vi "SetDG with FileParamters.vi"(8 "error in (no error)":errorcluster, 10 "State":T1, 11 "BME_DG_Base in":refnum<class "BME_DG_Base.lvclass">) -> (0 "error out":errorcluster, 3 "BME_DG_Base out":refnum<class "BME_DG_Base.lvclass">)   [LabVIEW 2009, in "BME_DG_Base.lvclass"]
uses:
  BME_DG_Base.lvclass
  LV-BME Interface/Typedefs For ReadParameters()/BME_DG_BME_State.ctl
  LV-BME Interface/Typedefs For ReadParameters()/BME_DG_DelayChannelData.ctl
  BME_DG_Base.lvclass/BME_DG_Base.ctl
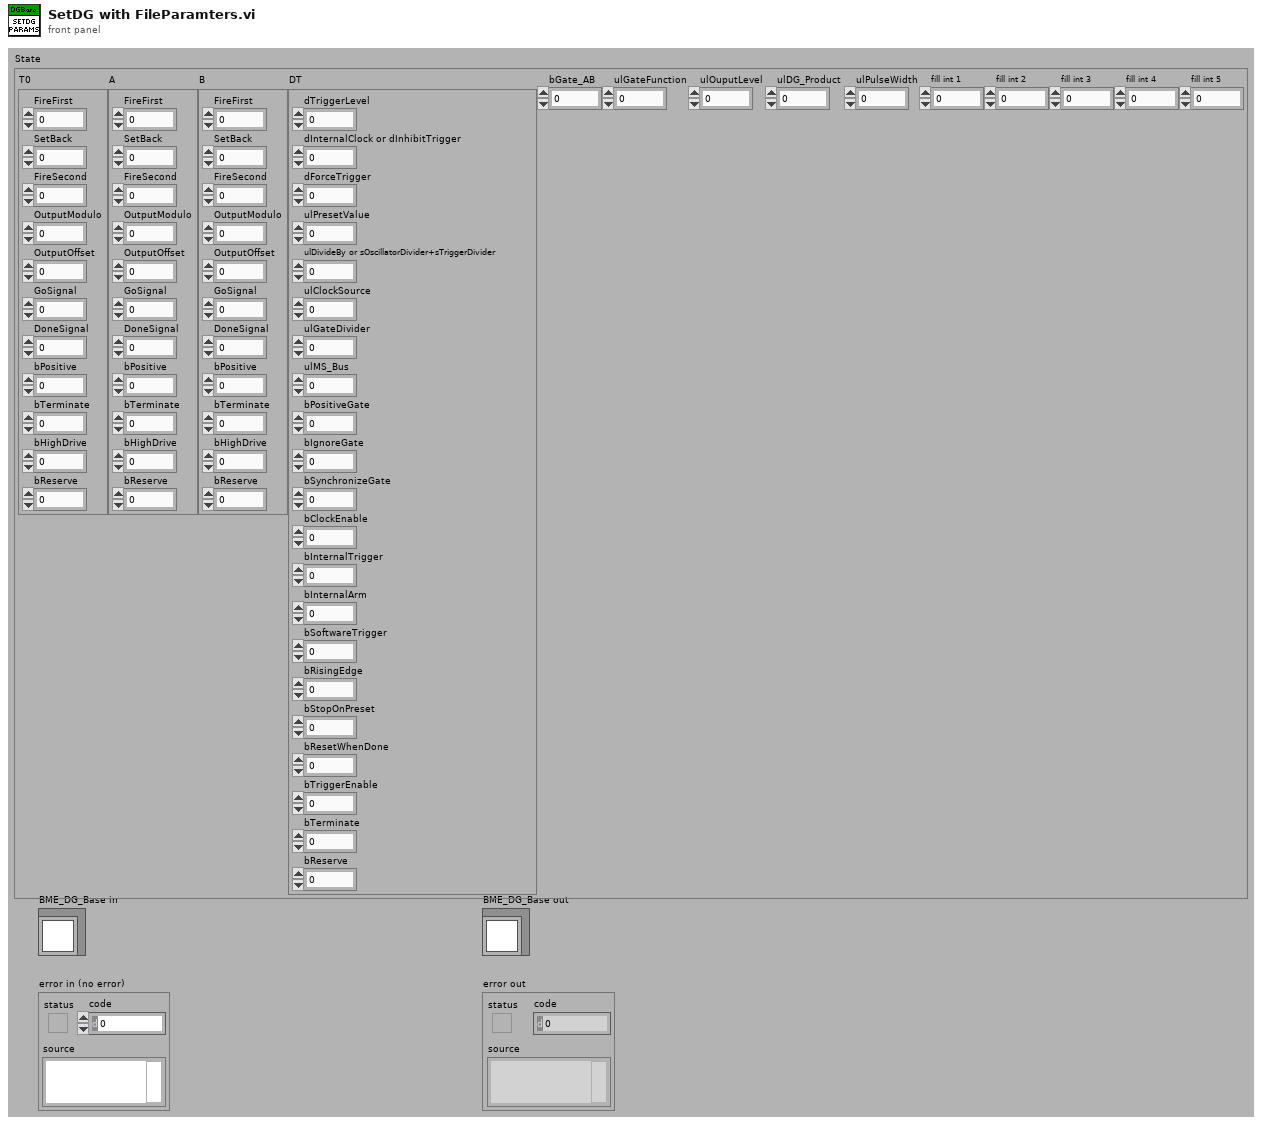
[diagram p1: front panel]
types:
  T1 = typedef "BME_DG_BME_State.ctl" = cluster{"T0":T2, "A":T2, "B":T2, "DT":cluster{"dTriggerLevel":dbl, "dInternalClock or dInhibitTrigger":dbl, "dForceTrigger":dbl, "ulPresetValue":u32, "ulDivideBy or sOscillatorDivider+sTriggerDivider":u32, "ulClockSource":u32, "ulGateDivider":u32, "ulMS_Bus":u32, "bPositiveGate":u32, "bIgnoreGate":u32, "bSynchronizeGate":u32, "bClockEnable":u32, "bInternalTrigger":u32, "bInternalArm":u32, "bSoftwareTrigger":u32, "bRisingEdge":u32, "bStopOnPreset":u32, "bResetWhenDone":u32, "bTriggerEnable":u32, "bTerminate":u32, "bReserve":u32}, "bGate_AB":u32, "ulGateFunction":u32, "ulOuputLevel":u32, "ulDG_Product":u32, "ulPulseWidth":u32, "fill int 1":i32, "fill int 2":i32, "fill int 3":i32, "fill int 4":i32, "fill int 5":i32}
  T2 = typedef "BME_DG_DelayChannelData.ctl" = cluster{"FireFirst":dbl, "SetBack":dbl, "FireSecond":dbl, "OutputModulo":u32, "OutputOffset":u32, "GoSignal":u32, "DoneSignal":u32, "bPositive":u32, "bTerminate":u32, "bHighDrive":u32, "bReserve":u32}
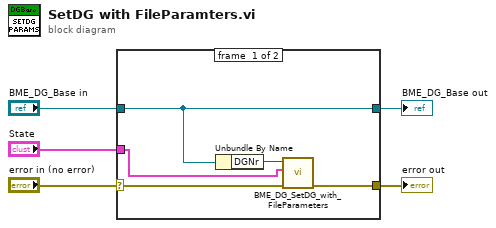
[diagram p0: block diagram]
diagram:
  n1 = case shown="No Error" "error in (no error)" {
    selector: "error in (no error)" -> [w8 w12]
    tunnel: [w7 w12] -> w4
    tunnel: [w10 w11] -> w2
    tunnel: "BME_DG_Base in" -> [w10 w11]
    tunnel: "State" -> [w6 _]
    frame #0 {
      n2 = Unbundle By Name(w10) -> ("DGNr"=w9:i32)
      n3 = call "BME_DG_SetDG_with_FileParameters.vi"("error in (no error)"=w8, "State"=w6, "DG_Number"=w9) -> ("error out"=w7:errorcluster)  [unwired: 7 in, 1 out]
    }
    frame #1 {
    }
  }
  "error out" <- w4
  "BME_DG_Base out" <- w2
